vi "Pockels Cal-Prevention message.vi"() -> (3 "Cancel":bool)   [LabVIEW 2020]
uses:
  Globals/gl_Calibration globals.vi
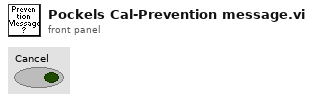
[diagram p1: front panel]
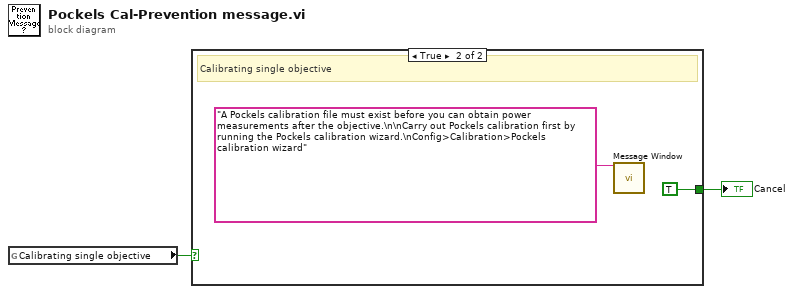
[diagram p0: block diagram]
diagram:
  n1 = global read "gl_Calibration globals.vi" "Calibrating single objective"() -> (w2:bool)
  n2 = case shown="True" w2 {
    tunnel: [_ TRUE] -> w1
    frame False {
    }
    frame True {
      # "Calibrating single objective"
      n3 = call "Message Window.vi"("Message string"="A Pockels calibration file must exist before you can obtain power measurements after the objective.\n\nCarry out Pockels calibration first by running the Pockels calibration wizard.\nConfig>Calibration>Pockels calibration wizard") -> ()  [unwired: 10 in, 1 out]
    }
  }
  "Cancel" <- w1
